vi "format_coords_str(new).vi"(2 "DEC str":string, 4 "RA str":string) -> (0 "%s DEC":string, 1 "%s RA":string)   [LabVIEW 2019]
panel:
  out "String 2":string
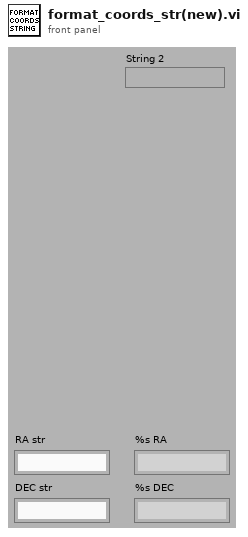
[diagram p1: front panel]
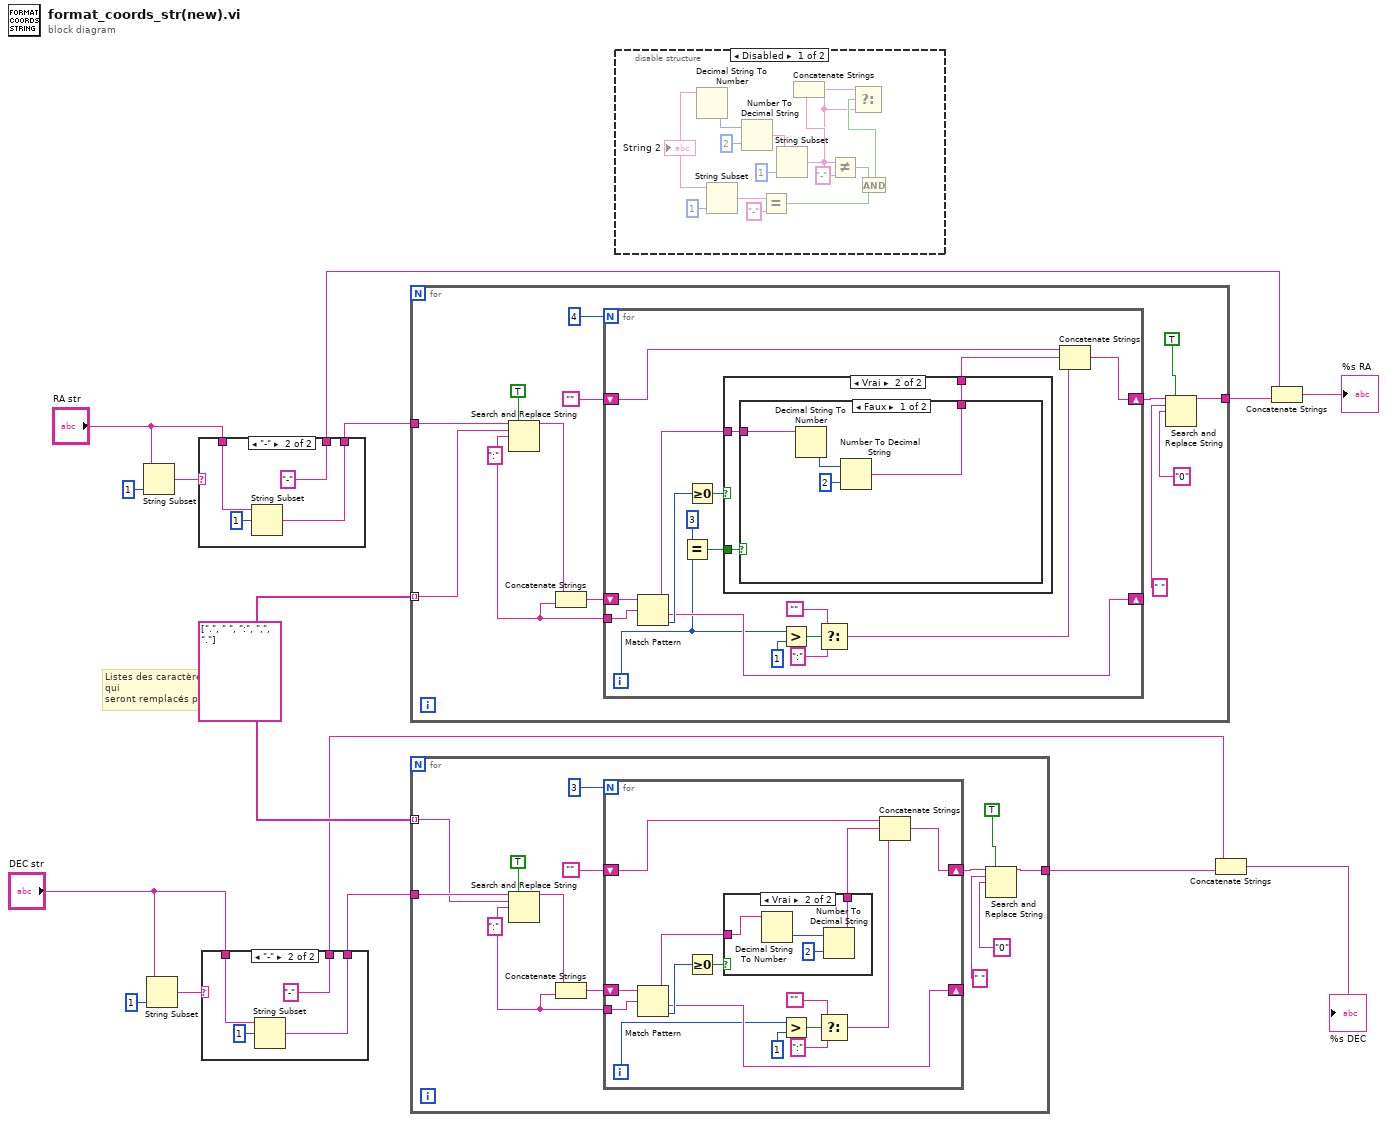
[diagram p0: block diagram]
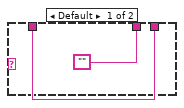
[diagram p2: hidden frame]
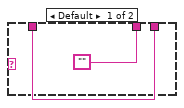
[diagram p3: hidden frame]
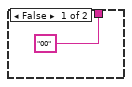
[diagram p5: hidden frame]
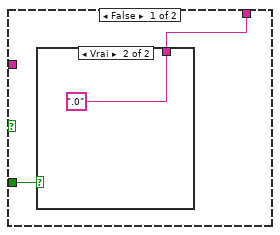
[diagram p6: hidden frame]
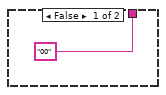
[diagram p7: hidden frame]
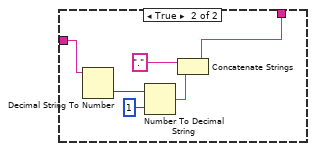
[diagram p8: hidden frame]
diagram:
  w15 = string[] [".", " ", ":", ",", "."] ("Array")
  # "Listes des caractères qui\nseront remplacés par \":\""
  n1 = String Subset(string="RA str", length (rest)=1 ("length (rest)")) -> (substring=w13:string)  [unwired: 1 in]
  n2 = String Subset(string="DEC str", length (rest)=1 ("length (rest)")) -> (substring=w7:string)  [unwired: 1 in]
  n3 = case shown="\"-\"" w13 {
    tunnel: "RA str" -> [w17 w21]
    tunnel: [w17 w19] -> w11
    tunnel: ["" "-"] -> w8
    frame Default {
    }
    frame "-" {
      n4 = String Subset(string=w21, offset (0)=1) -> (substring=w19:string)  [unwired: 1 in]
    }
  }
  n5 = case shown="\"-\"" w7 {
    tunnel: "DEC str" -> [w23 w27]
    tunnel: [w23 w25] -> w4
    tunnel: ["" "-"] -> w1
    frame Default {
    }
    frame "-" {
      n6 = String Subset(string=w27, offset (0)=1) -> (substring=w25:string)  [unwired: 1 in]
    }
  }
  n7 = for {
    tunnel: [w40] -> w9
    tunnel: w11 -> [w39]
    tunnel: w15 -> [w38] mode=indexing
    w31 = ":" ("replace string (\"\")")
    n8 = Search and Replace String(replace all?=TRUE ("replace all? (F)"), input string=w39, search string=w38, replace string=w31) -> (result string=w33:string)  [unwired: 4 in, 3 out]
    n9 = Concatenate Strings(w33, w31) -> (w34:string)
    n10 = for {
      N: 4 -> [_]
      shift-right: [w53] -> _
      shift-left: w34 -> [w56]
      shift-right: [w57] -> w32
      shift-left: "" -> [w51]
      tunnel: w31 -> [w49]
      i -> [w42]
      n11 = Match Pattern(string=w56, regular expression=w49) -> (before substring=w52:string, after substring=w53:string, offset past match=w54:i32)  [unwired: 1 in, 1 out]
      n12 = Equal?(x=3, y=w42) -> (x = y?=w43:bool)
      n13 = Greater Or Equal To 0?(x=w54) -> (x >= 0?=w55:bool)
      n14 = case shown="Vrai" w55 {
        tunnel: w52 -> [_ w64]
        tunnel: [w59 w63] -> w50
        tunnel: w43 -> [w58 w62]
        frame False {
          n15 = case shown="Vrai" w58 {
            tunnel: ["00" ".0"] -> w59
            frame False {
            }
            frame True {
            }
          }
        }
        frame True {
          n16 = case shown="Faux" w62 {
            tunnel: w64 -> [w66 w72]
            tunnel: [w65 w69] -> w63
            frame False {
              n17 = Decimal String To Number(string=w66) -> (number=w67:i32)  [unwired: 2 in, 1 out]
              n18 = Number To Decimal String(number=w67, width (-)=i16 2) -> (decimal integer string=w65:string)
            }
            frame True {
              n19 = Decimal String To Number(string=w72) -> (number=w73:i32)  [unwired: 2 in, 1 out]
              n20 = Number To Decimal String(number=w73, width (-)=i16 1) -> (decimal integer string=w71:string)
              n21 = Concatenate Strings(".", w71) -> (w69:string)
            }
          }
        }
      }
      n22 = Greater?(x=w42, y=1) -> (0:w47:bool)
      n23 = Select(t="", s=w47, f=":" ("replace string (\"\")")) -> (s? t:f=w44:string)
      n24 = Concatenate Strings(w51, w50, w44) -> (w57:string)
    }
    n25 = Search and Replace String(replace all?=TRUE ("replace all? (F)"), input string=w32, search string=" ", replace string="0" ("replace string (\"\")")) -> (result string=w40:string)  [unwired: 4 in, 3 out]
  }
  n26 = for {
    tunnel: [w87] -> w3
    tunnel: w4 -> [w86]
    tunnel: w15 -> [w85] mode=indexing
    w78 = ":" ("replace string (\"\")")
    n27 = Search and Replace String(replace all?=TRUE ("replace all? (F)"), input string=w86, search string=w85, replace string=w78) -> (result string=w80:string)  [unwired: 4 in, 3 out]
    n28 = Concatenate Strings(w80, w78) -> (w81:string)
    n29 = for {
      N: 3 -> [_]
      shift-right: [w98] -> _
      shift-left: w81 -> [w101]
      shift-right: [w102] -> w79
      shift-left: "" -> [w96]
      tunnel: w78 -> [w94]
      i -> [w89]
      n30 = Match Pattern(string=w101, regular expression=w94) -> (before substring=w97:string, after substring=w98:string, offset past match=w99:i32)  [unwired: 1 in, 1 out]
      n31 = Greater Or Equal To 0?(x=w99) -> (x >= 0?=w100:bool)
      n32 = case shown="Vrai" w100 {
        tunnel: w97 -> [_ w105]
        tunnel: ["00" w104] -> w95
        frame False {
        }
        frame True {
          n33 = Decimal String To Number(string=w105) -> (number=w106:i32)  [unwired: 2 in, 1 out]
          n34 = Number To Decimal String(number=w106, width (-)=i16 2) -> (decimal integer string=w104:string)
        }
      }
      n35 = Greater?(x=w89, y=1) -> (0:w92:bool)
      n36 = Select(t="", s=w92, f=":" ("replace string (\"\")")) -> (s? t:f=w88:string)
      n37 = Concatenate Strings(w96, w95, w88) -> (w102:string)
    }
    n38 = Search and Replace String(replace all?=TRUE ("replace all? (F)"), input string=w79, search string=" ", replace string="0" ("replace string (\"\")")) -> (result string=w87:string)  [unwired: 4 in, 3 out]
  }
  n39 = disable-structure shown="Disabled" {
    frame Disabled {
      w120 = "-"
      n40 = Decimal String To Number() -> (string=w110:string, number=w109:i32)  [unwired: 2 in, 1 out]
      "String 2" <- w110
      n41 = String Subset(string=w110, length (rest)=1 ("length (rest)")) -> (substring=w112:string)  [unwired: 1 in]
      n42 = Number To Decimal String(number=w109, width (-)=i16 2) -> (decimal integer string=w115:string)
      n43 = Equal?(x=w112, y="-") -> (x = y?=w117:bool)
      n44 = String Subset(string=w115, length (rest)=1 ("length (rest)")) -> (substring=w119:string)  [unwired: 1 in]
      n45 = Concatenate Strings(w119, w120) -> (w118:string)
      n46 = Not Equal?(x=w119, y=w120) -> (x != y?=w116:bool)
      n47 = And(x=w116, y=w117) -> (x .and. y?=w121:bool)
      n48 = Select(t=w118, s=w121, f=w119) -> ()  [unwired: 1 out]
    }
    frame Enabled {
    }
  }
  n49 = Concatenate Strings(w1, w3) -> (→"%s DEC":string)
  n50 = Concatenate Strings(w8, w9) -> (→"%s RA":string)
